vi "ProyectoFinal.vi"() -> ()   [LabVIEW 2020]
uses:
  <vilib>/Instr/_visa.llb/VISA Configure Serial Port (Instr).vi
panel:
  in  "Accionar Dispensador":bool
  in  "Accionar Bomba":bool
  out "String 7":string
  out "String 6":string
  out "String 5":string
  out "String 4":string
  out "String 3":string
  out "String 2":string
  out "String":string
  in  "Cerrar Sesión":bool
  out "Nombre confirmado":string
  out "Confirmado":bool
  in  "Contraseña":string
  in  "Nombre":string
  out "x .and. y?":bool
  in  "Minuto":dbl min=0.0 max=59.0 step=1.0
  in  "Hora":dbl min=0.0 max=12.0 step=1.0
  out "Hora":string
  out "Nivel":dbl
  out "Bomba":bool
  in  "ValorMenorNivel":dbl=19.0 min=15.0 max=19.0 step=1.0
  in  "ValorMayorNivel":dbl=50.0 min=50.0 max=90.0 step=1.0
  out "Calentador":bool
  in  "ValorMenorTemp":dbl=25.0
  in  "ValorMayorTemp":dbl=27.0 min=20.0 max=30.0 step=1.0
  out "Temperatura":dbl
  in  "stop":bool
  in  "VISA resource name":refnum<visa-resource-name>
  # "PECERA AUTOMATIZADA"
  # "PUERTO ARDUINO"
  # "ACTUADORES"
  # "INDICADORES"
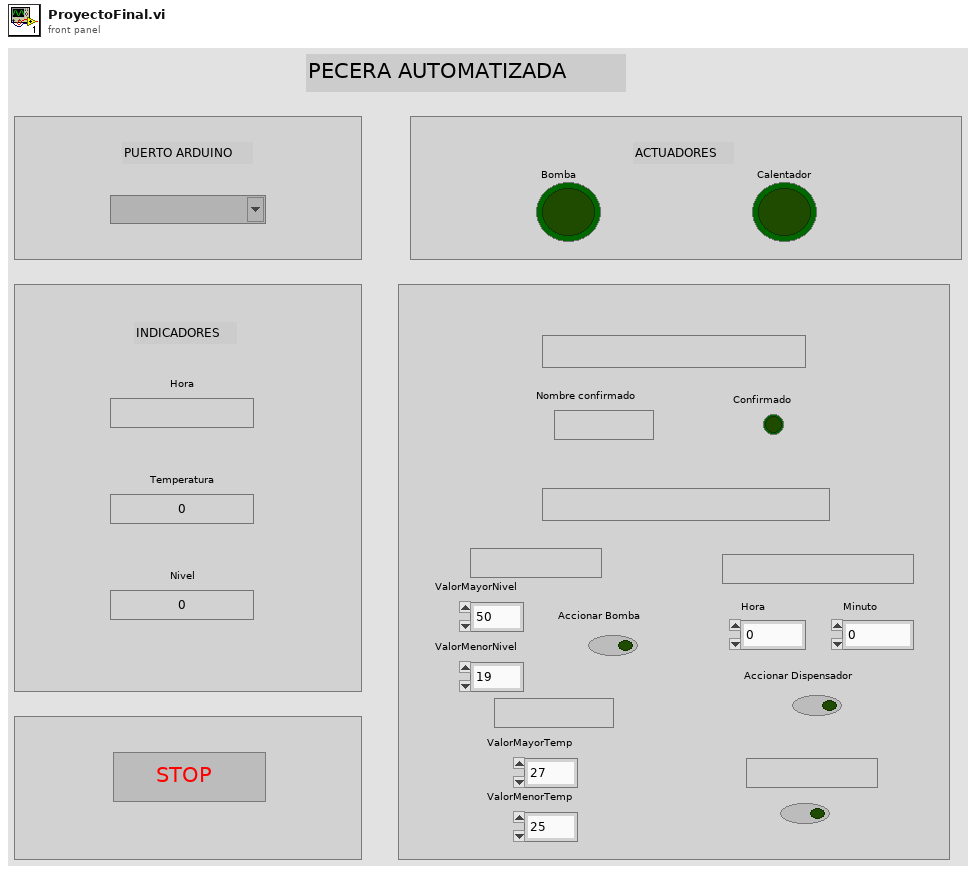
[diagram p1: front panel]
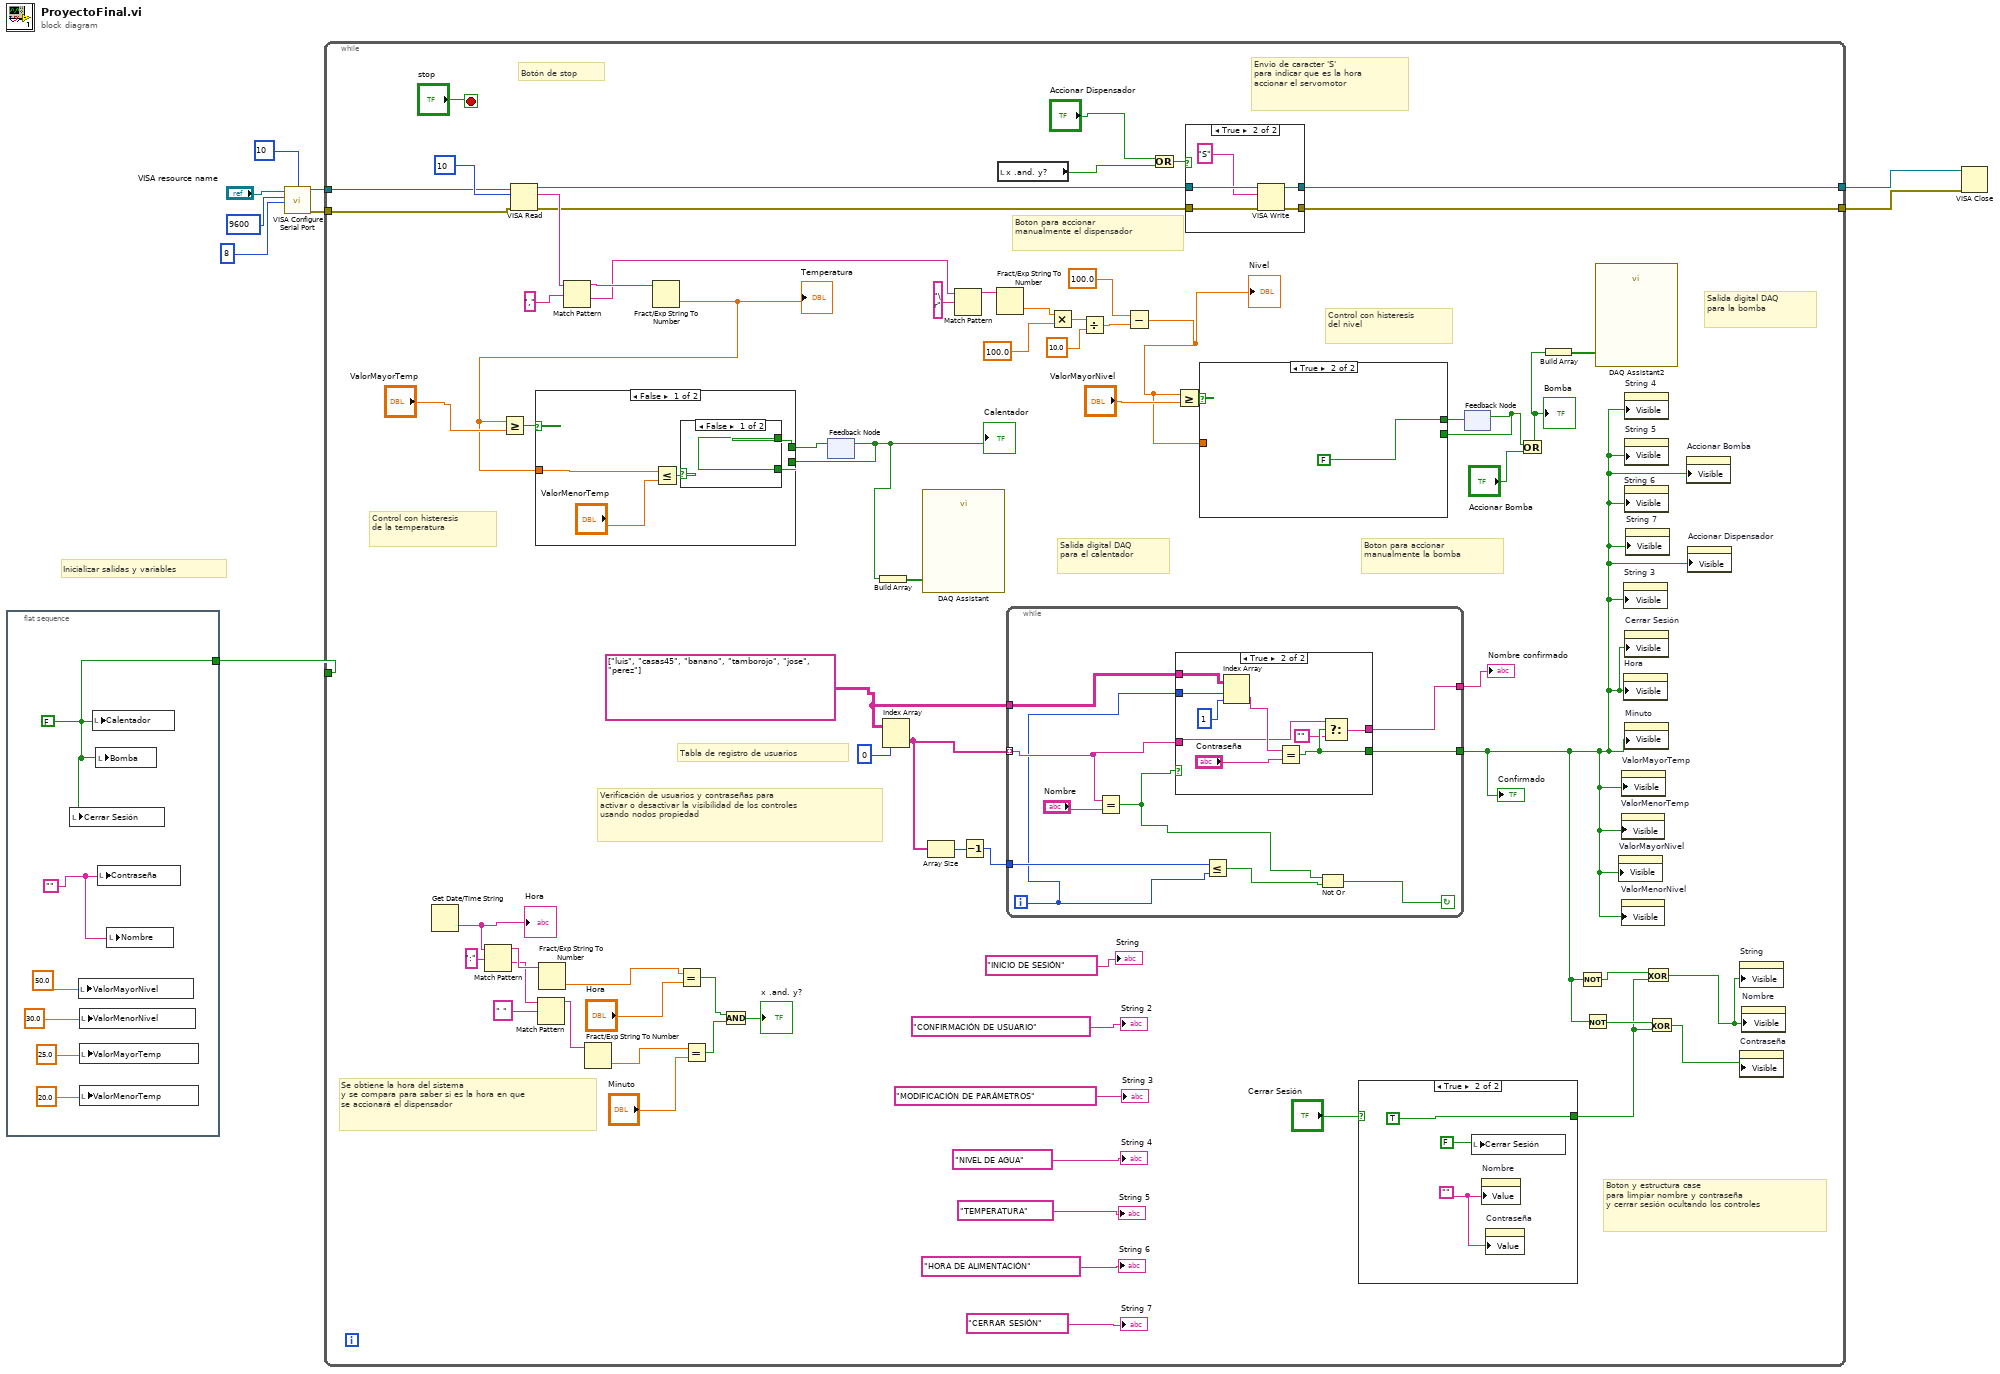
[diagram p0: block diagram]
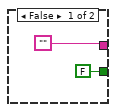
[diagram p3: hidden frame]
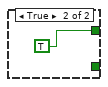
[diagram p4: hidden frame]
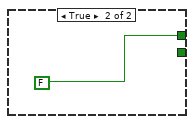
[diagram p5: hidden frame]
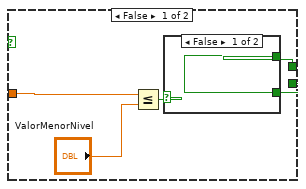
[diagram p7: hidden frame]
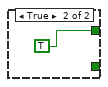
[diagram p8: hidden frame]
diagram:
  # "Inicializar salidas y variables"
  n1 = flat-sequence {
    tunnel: [w14] -> w1
    frame #0 {
      w15 = ""
      w14 = FALSE
      n2 = local write "Cerrar Sesión"(w14) -> ()
      n3 = local write "ValorMayorNivel"(50.0) -> ()
      n4 = local write "ValorMenorNivel"(30.0) -> ()
      n5 = local write "ValorMayorTemp"(25.0) -> ()
      n6 = local write "ValorMenorTemp"(20.0) -> ()
      n7 = local write "Calentador"(w14) -> ()
      n8 = local write "Bomba"(w14) -> ()
      n9 = local write "Contraseña"(w15) -> ()
      n10 = local write "Nombre"(w15) -> ()
    }
  }
  n11 = call-poly "VISA Configure Serial Port"("VISA resource name"="VISA resource name", "termination char\n(0xA = '\\n' = LF)"=u8 10 ("termination char\n(0xA = '\\n' = LF)"), "baud rate (9600)"=u32 9600, "data bits (8)"=u16 8) -> ("VISA resource name out"=w9:refnum<visa-resource-name>, "error out"=w4:errorcluster)  [unwired: 10 in]
  n12 = while {
    tunnel: w9 -> [w83]
    tunnel: w4 -> [w82]
    tunnel: [w69] -> w3
    tunnel: [w70] -> w2
    tunnel: w1 -> [_]
    stop <- "stop" stop-if-true
    w48 = string[][] [["luis", "casas45"], ["banano", "tamborojo"], ["jose", "perez"]]
    # "Boton y estructura case\npara limpiar nombre y contraseña\ny cerrar sesión ocultando los controles"
    # "Salida digital DAQ\npara la bomba"
    # "Salida digital DAQ\npara el calentador"
    # "Botón de stop"
    # "Boton para accionar\nmanualmente el dispensador"
    # "Boton para accionar\nmanualmente la bomba"
    # "Control con histeresis\ndel nivel"
    # "Control con histeresis\nde la temperatura"
    # "Verificación de usuarios y contraseñas para\nactivar o desactivar la visibilidad de los controles\nusando nodos propiedad"
    # "Se obtiene la hora del sistema\ny se compara para saber si es la hora en que\nse accionará el dispensador"
    # "Tabla de registro de usuarios"
    # "Envio de caracter 'S'\npara indicar que es la hora\naccionar el servomotor"
    n13 = Get Date/Time String() -> (time string=w68:string)  [unwired: 3 in, 1 out]
    "Hora" <- w68
    n14 = Match Pattern(string=w68, regular expression=":") -> (before substring=w66:string, after substring=w63:string)  [unwired: 1 in, 2 out]
    n15 = VISA Read(VISA resource name=w83, byte count=u32 10, error in (no error)=w82) -> (VISA resource name out=w72:refnum<visa-resource-name>, read buffer=w81:string, error out=w71:errorcluster)  [unwired: 1 out]
    n16 = Match Pattern(string=w63, regular expression=" ") -> (before substring=w64:string)  [unwired: 1 in, 3 out]
    n17 = Fract/Exp String To Number(string=w66) -> (number=w62:dbl)  [unwired: 3 in, 1 out]
    n18 = Match Pattern(string=w81, regular expression=",") -> (before substring=w79:string, after substring=w77:string)  [unwired: 1 in, 2 out]
    n19 = Fract/Exp String To Number(string=w64) -> (number=w61:dbl)  [unwired: 3 in, 1 out]
    n20 = Fract/Exp String To Number(string=w79) -> (number=w37:dbl)  [unwired: 3 in, 1 out]
    "Temperatura" <- w37
    n21 = Greater Or Equal?(x=w37, y="ValorMayorTemp") -> (x >= y?=w55:bool)
    n22 = Equal?(x=w62, y="Hora") -> (x = y?=w58:bool)
    n23 = Equal?(x=w61, y="Minuto") -> (x = y?=w57:bool)
    n24 = And(x=w58, y=w57) -> (x .and. y?=→"x .and. y?":bool)
    n25 = feedback #1() -> (w24:bool)  [unwired: 1 in]
    "Calentador" <- w24
    n26 = case shown="False" w55 {
      tunnel: w37 -> [w114 _]
      tunnel: [w112 FALSE] -> w54
      tunnel: w24 -> [w111 _]
      frame False {
        n27 = Less Or Equal?(x=w114, y="ValorMenorTemp") -> (x <= y?=w113:bool)
        n28 = case shown="False" w113 {
          tunnel: [w115 TRUE] -> w112
          tunnel: w111 -> [w115 _]
          frame False {
          }
          frame True {
          }
        }
      }
      frame True {
      }
    }
    n29 = feedback-in #1(w54) -> ()
    n30 = Build Array(w24) -> (w25:bool[])
    n31 = Index Array "Index Array"(array=w48, index (col)=0 ("disabled index (col)")) -> (element=w51:string[])  [unwired: 1 in]
    n32 = call "DAQ Assistant"("data"=w25) -> ()  [unwired: 17 in, 2 out]
    n33 = Array Size(array=w51) -> (size(s)=w49:i32)
    n34 = Match Pattern(string=w77, regular expression="\r") -> (before substring=w76:string)  [unwired: 1 in, 3 out]
    n35 = Decrement(x=w49) -> (x-1=w50:i32)
    n36 = Fract/Exp String To Number(string=w76) -> (number=w31:dbl)  [unwired: 3 in, 1 out]
    n37 = local read "x .and. y?"() -> (w21:bool)
    n38 = while {
      tunnel: w50 -> [w96]
      tunnel: w51 -> [w94] mode=indexing
      tunnel: [w93] -> w16
      tunnel: [w92] -> w52
      tunnel: w48 -> [w91]
      i -> [w90]
      stop <- w98 continue-if-true
      n39 = Equal?(x=w94, y="Nombre") -> (x = y?=w89:bool)
      n40 = case shown="True" w89 {
        tunnel: w91 -> [_ w103]
        tunnel: w94 -> [_ w106]
        tunnel: [FALSE w105] -> w93
        tunnel: ["" w104] -> w92
        tunnel: w90 -> [_ w102]
        frame False {
        }
        frame True {
          n41 = Index Array(array=w103, index (row)=w102, index (col)=1) -> (element=w107:string)
          n42 = Equal?(x=w107, y="Contraseña") -> (x = y?=w105:bool)
          n43 = Select(t=w106, s=w105, f="") -> (s? t:f=w104:string)
        }
      }
      n44 = Less Or Equal?(x=w96, y=w90) -> (x <= y?=w97:bool)
      n45 = Not Or(1:w97, 2:w89) -> (0:w98:bool)
    }
    "Confirmado" <- w16
    "Nombre confirmado" <- w52
    n46 = Multiply(x=w31, y=100.0) -> (x*y=w30:dbl)
    n47 = Divide(x=w30, y=10.0) -> (x/y=w28:dbl)
    n48 = Subtract(x=100.0, y=w28) -> (x-y=w26:dbl)
    "Nivel" <- w26
    n49 = Or(x="Accionar Dispensador", y=w21) -> (x .or. y?=w22:bool)
    n50 = Greater Or Equal?(x=w26, y="ValorMayorNivel") -> (x >= y?=w75:bool)
    n51 = case shown="True" w22 {
      tunnel: w72 -> [w119 w123]
      tunnel: w71 -> [w118 w124]
      tunnel: [w119 w122] -> w70
      tunnel: [w118 w121] -> w69
      frame False {
      }
      frame True {
        n52 = VISA Write(VISA resource name=w123, write buffer="S", error in (no error)=w124) -> (VISA resource name out=w122:refnum<visa-resource-name>, error out=w121:errorcluster)  [unwired: 1 out]
      }
    }
    n53 = case shown="True" "Cerrar Sesión" {
      tunnel: [_ TRUE] -> w43
      frame False {
      }
      frame True {
        w86 = ""
        n54 = local write "Cerrar Sesión"(FALSE) -> ()
        n55 = property on="Nombre" class="Str"("Value"=w86) -> ()  [unwired: 2 in, 2 out]
        n56 = property on="Contraseña" class="Str"("Value"=w86) -> ()  [unwired: 2 in, 2 out]
      }
    }
    n57 = feedback #2() -> (w17:bool)  [unwired: 1 in]
    n58 = case shown="True" w75 {
      tunnel: w26 -> [w129 _]
      tunnel: [w127 FALSE] -> w74
      tunnel: w17 -> [w126 _]
      frame False {
        n59 = Less Or Equal?(x=w129, y="ValorMenorNivel") -> (x <= y?=w128:bool)
        n60 = case shown="False" w128 {
          tunnel: [w130 TRUE] -> w127
          tunnel: w126 -> [w130 _]
          frame False {
          }
          frame True {
          }
        }
      }
      frame True {
      }
    }
    n61 = feedback-in #2(w74) -> ()
    n62 = Or(x=w17, y="Accionar Bomba") -> (x .or. y?=w18:bool)
    "Bomba" <- w18
    n63 = Build Array(w18) -> (w23:bool[])
    n64 = Not(x=w16) -> (.not. x?=w45:bool)
    n65 = Not(x=w16) -> (.not. x?=w44:bool)
    n66 = call "DAQ Assistant2"("data"=w23) -> ()  [unwired: 17 in, 2 out]
    n67 = property on="ValorMayorNivel" class="DigNum (strict)"("Visible"=w16) -> ()  [unwired: 2 in, 2 out]
    n68 = property on="ValorMenorTemp" class="DigNum (strict)"("Visible"=w16) -> ()  [unwired: 2 in, 2 out]
    n69 = property on="ValorMenorNivel" class="DigNum (strict)"("Visible"=w16) -> ()  [unwired: 2 in, 2 out]
    n70 = property on="ValorMayorTemp" class="DigNum (strict)"("Visible"=w16) -> ()  [unwired: 2 in, 2 out]
    n71 = property on="String 3" class="Str"("Visible"=w16) -> ()  [unwired: 2 in, 2 out]
    n72 = property on="Hora" class="DigNum (strict)"("Visible"=w16) -> ()  [unwired: 2 in, 2 out]
    n73 = property on="String 4" class="Str"("Visible"=w16) -> ()  [unwired: 2 in, 2 out]
    n74 = property on="String 5" class="Str"("Visible"=w16) -> ()  [unwired: 2 in, 2 out]
    n75 = property on="String 6" class="Str"("Visible"=w16) -> ()  [unwired: 2 in, 2 out]
    n76 = property on="Cerrar Sesión" class="Bool (strict)"("Visible"=w16) -> ()  [unwired: 2 in, 2 out]
    n77 = property on="Minuto" class="DigNum (strict)"("Visible"=w16) -> ()  [unwired: 2 in, 2 out]
    n78 = property on="String 7" class="Str"("Visible"=w16) -> ()  [unwired: 2 in, 2 out]
    n79 = Exclusive Or(1:w43, 2:w45) -> (0:w40:bool)
    n80 = Exclusive Or(1:w43, 2:w44) -> (0:w46:bool)
    n81 = property on="Accionar Bomba" class="Bool (strict)"("Visible"=w16) -> ()  [unwired: 2 in, 2 out]
    n82 = property on="Accionar Dispensador" class="Bool (strict)"("Visible"=w16) -> ()  [unwired: 2 in, 2 out]
    n83 = property on="String" class="Str"("Visible"=w40) -> ()  [unwired: 2 in, 2 out]
    n84 = property on="Contraseña" class="Str"("Visible"=w46) -> ()  [unwired: 2 in, 2 out]
    n85 = property on="Nombre" class="Str"("Visible"=w40) -> ()  [unwired: 2 in, 2 out]
    "String" <- "INICIO DE SESIÓN"
    "String 2" <- "CONFIRMACIÓN DE USUARIO"
    "String 3" <- "MODIFICACIÓN DE PARÁMETROS"
    "String 5" <- "TEMPERATURA"
    "String 7" <- "CERRAR SESIÓN"
    "String 6" <- "HORA DE ALIMENTACIÓN"
    "String 4" <- "NIVEL DE AGUA"
  }
  n86 = VISA Close(VISA resource name=w2, error in (no error)=w3) -> ()  [unwired: 1 out]
